vi "Neocera Range to Watts.vi"(10 "Maximum current":dbl=1.0, 11 "Integer range":i32) -> (2 "Heater off":bool, 3 "Watts":dbl format="%#_6p")   [LabVIEW 2015]
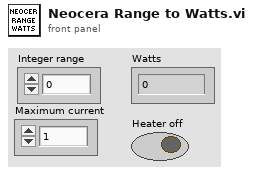
[diagram p1: front panel]
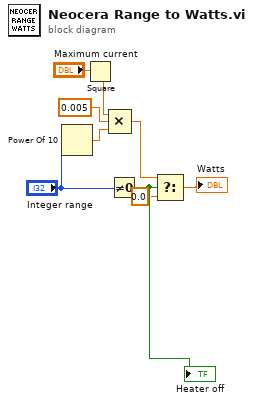
[diagram p0: block diagram]
diagram:
  n1 = Power Of 10(x="Integer range") -> (10^x=w3:dbl)
  n2 = Square(x="Maximum current") -> (x^2=w1:dbl)
  n3 = Compound Arithmetic op=MULTIPLY(w1, 0.005, w3) -> (w6:dbl)
  n4 = Not Equal To 0?(x="Integer range") -> (x != 0?=w9:bool)
  "Heater off" <- w9
  n5 = Select(t=w6, s=w9, f=0.0) -> (s? t:f=→"Watts":dbl)
